vi "Main.vi"(11 "Module Admin":refnum<class "Delacor_lib_QMH_Module Admin.lvclass">) -> ()   [LabVIEW 2021, in "SCOPE.lvlib"]
doc: "This template is based off of the Queued Message Handler design pattern and the Queued Message Handler project template that ships with LabVIEW.\n\nThe main difference is that the queue is private to this module and communication between modules is performed via Broadcast and Request events.\n\nRequest events are wrapped in public API methods and are handled in the Event Handling Loop (EHL) of this VI. Any module can register for Broadcast events sent by this module. The EHL generates messages based on user interface actions.\n\nThe Message Handling Loop (MHL) processes messages generated by the EHL, or by other messages. The messages are string values, so new messages can be added easily to the Message Cases case structure in the MHL. Each message cluster can also provide an optional value for Message Data, which is a variant that can be converted to whatever message-specific data is required.\n_____\nBased on Delacor QMH Project Template 5.0.0.82.\n\n<b>Note:</b> This VI was modified by the <b>Validate DQMH Module</b> tool to add a 'Panel Hidden' status updated broadcast to the Panel Close? event when External Launch = TRUE.\n\n<b>Note:</b> This VI was modified by the <b>Validate DQMH Module</b> tool to add a call to the Error Reported VI at the end of the 'Exit' MHL frame.\n\n<b>Note:</b> This VI was modified by the <b>Validate DQMH Module</b> tool to wrap the FP.Open method in the module close code with a Conditional Disable Structure so it does not execute when the Main VI is running as a built EXE."
uses:
  SCOPE.lvlib
  <vilib>/Delacor/Delacor QMH/Libraries/Module Admin_class/Delacor_lib_QMH_Module Admin.lvclass
  Module Data--cluster.ctl
  <vilib>/Delacor/Delacor QMH/Libraries/Message Queue_class/Delacor_lib_QMH_Message Queue.lvclass/Delacor_lib_QMH_Message Queue.ctl
  Stop Argument--cluster.ctl
  <vilib>/Delacor/Delacor QMH/Libraries/Module Admin_class/Delacor_lib_QMH_Module Admin.lvclass/Delacor_lib_QMH_Module Admin.ctl
  Simulation Argument--cluster.ctl
  Acquire Signal Argument--cluster.ctl
  Load in SubPane Argument--cluster.ctl
  UnLoad SubPane Argument--cluster.ctl
  <vilib>/Utility/miscctls.llb/LVPointTypeDef.ctl
  <vilib>/Delacor/Delacor QMH/Libraries/Message Queue_class/Delacor_lib_QMH_Enqueue Message (Single).vi
  <vilib>/Delacor/Delacor QMH/Libraries/Module Admin_class/Delacor_lib_QMH_Get External Launch.vi
  <vilib>/Utility/error.llb/Error Cluster From Error Code.vi
  <vilib>/ErrorRing/Error Ring.xnode
  <vilib>/Delacor/Delacor QMH/Libraries/Message Queue_class/Delacor_lib_QMH_Message Queue.lvclass
  Model/Model.lvlib
panel:
  in  "AcqTime":dbl=5.0
  out "ElapsedTime":dbl
  in  "Sim":bool
  out "WFM":dbl[](graph)
  in  "Acquire":bool
  out "Subpanel Ref":refnum<vi>
  out "ModuleName":string
  out "Sim?":bool
  in  "Simulate MHL Error":bool
  in  "Simulate EHL Error":bool
  out "error out":errorcluster
  out "Status":string
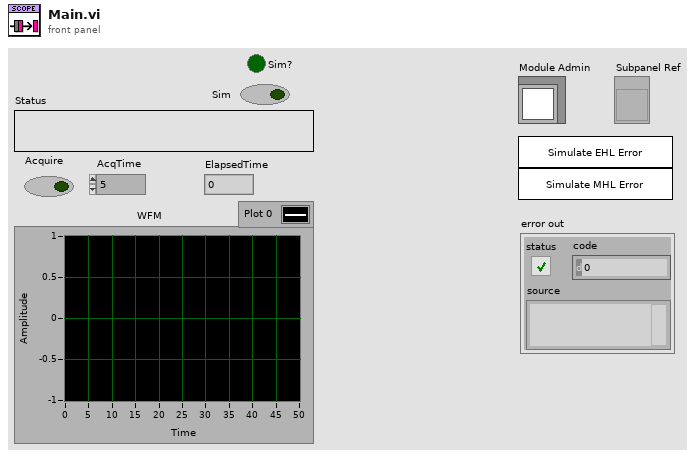
[diagram p1: front panel]
types:
  T1 = typedef "SCOPE.lvlib/Request Events--cluster.ctl" = cluster{"Stop Module":refnum<user-event>, "Show Panel":refnum<user-event>, "Hide Panel":refnum<user-event>, "Get Module Execution Status":refnum<user-event>, "Show Diagram":refnum<user-event>, "Simulation":refnum<user-event>, "Acquire Signal":refnum<user-event>, "Load in SubPane":refnum<user-event>, "UnLoad SubPane":refnum<user-event>}
  T2 = typedef "SCOPE.lvlib/Module Data--cluster.ctl" = cluster{"Status":string, "Sim":bool}
  T3 = enum32{"invalid lock state", "Not Locked", "Locked (No Password)", "Password-protected"}
  T4 = typedef "SCOPE.lvlib/Stop Argument--cluster.ctl" = cluster{"Origin":string, "Exit via Stop Module Req?":bool, "Wait for Module to stop?":bool}
  T5 = typedef "SCOPE.lvlib/Simulation Argument--cluster.ctl" = cluster{"Sim?":bool}
  T6 = typedef "SCOPE.lvlib/Acquire Signal Argument--cluster.ctl" = cluster{"Rate":i32, "AcqTime":dbl}
  T7 = typedef "SCOPE.lvlib/Load in SubPane Argument--cluster.ctl" = cluster{"Subpanel Ref":refnum<vi>}
  T8 = typedef "SCOPE.lvlib/UnLoad SubPane Argument--cluster.ctl" = cluster{"Subpanel Ref":refnum<vi>}
  T9 = typedef "LVPointTypeDef.ctl" = cluster{"Horizontal":i16, "Vertical":i16}
  T10 = enum32{"Invalid", "Standard", "Closed", "Hidden", "Minimized", "Maximized"}
  T11 = typedef "eventvkey.ctl" = enum16{"ASCII", "Enter", "Return", "Shift", "Ctrl", "Alt", "Cmd", "Opt", "Caps", "NumLock", "Clear", "Break", "Up", "Down", "Left", "Right", "Insert", "Delete", "Home", "End", "PageUp", "PageDown", "Escape", "Help", "Pause", "ScrollLock", "F1", "F2", "F3", "F4", "F5", "F6", "F7", "F8", "F9", "F10", "F11", "F12", "F13", "F14", "F15", "F16", "F17", "F18", "F19", "F20", "F21", "F22", "F23", "F24", "Play", "VolumeUp", "VolumeDown", "Mute", "Two Byte Char"}
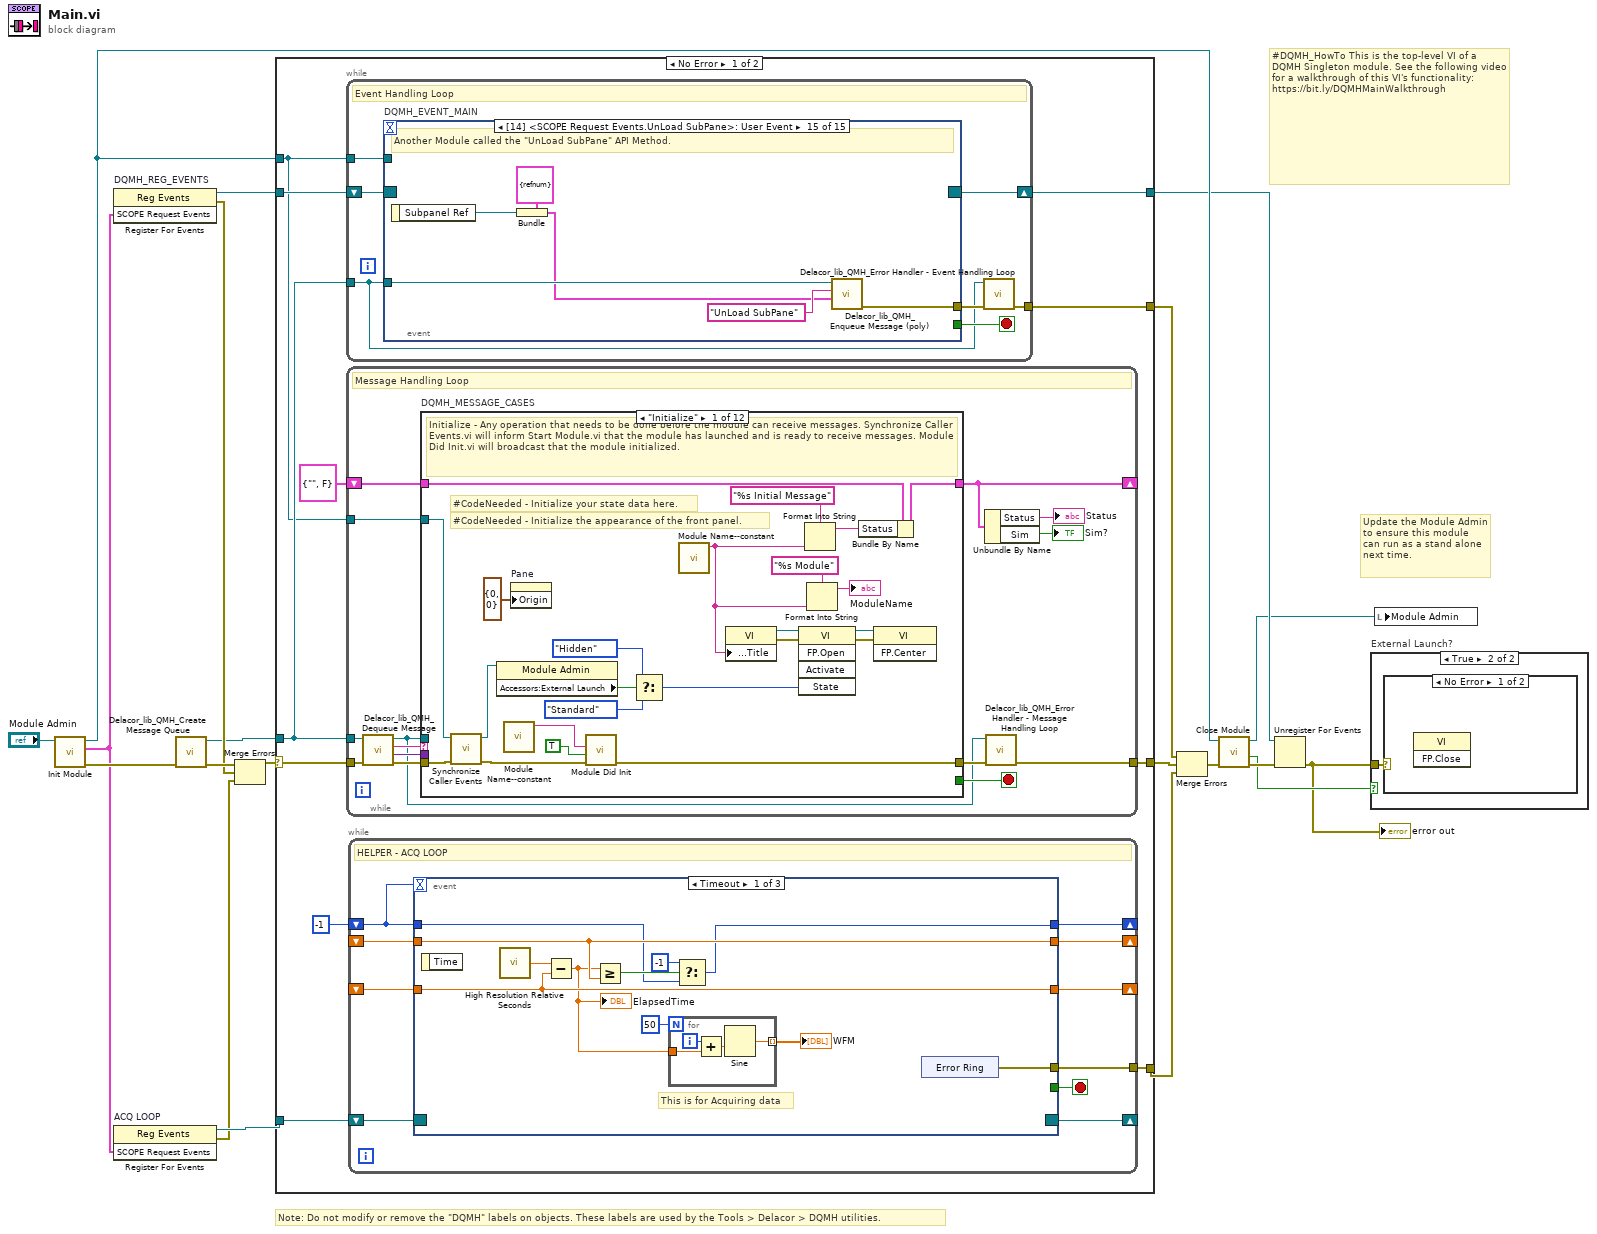
[diagram p0: block diagram]
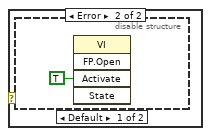
[diagram p3: hidden frame]
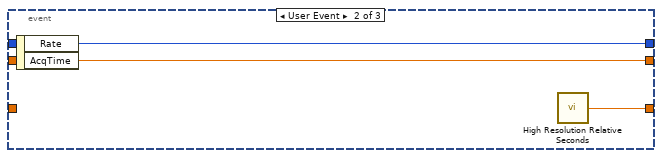
[diagram p5: hidden frame]
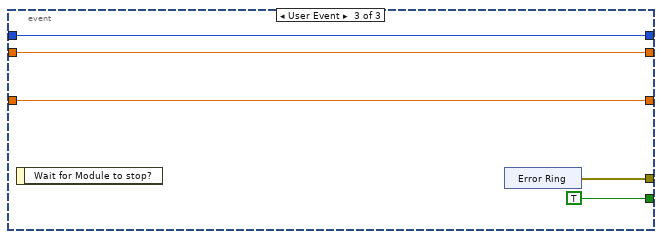
[diagram p6: hidden frame]
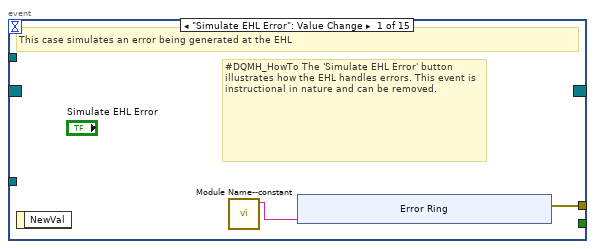
[diagram p7: hidden frame]
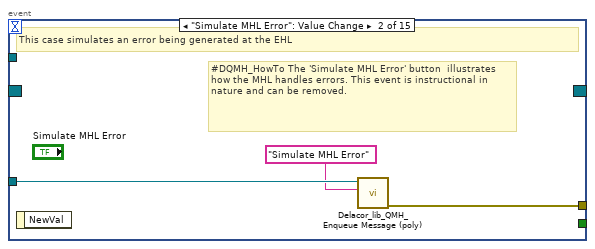
[diagram p8: hidden frame]
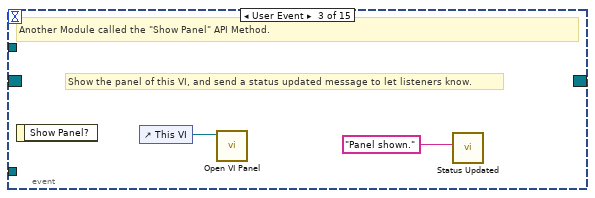
[diagram p9: hidden frame]
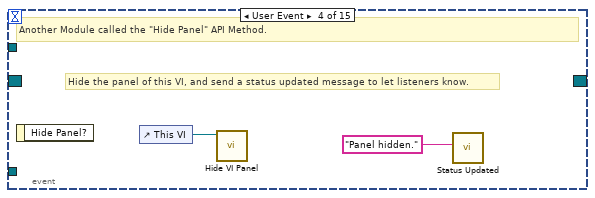
[diagram p10: hidden frame]
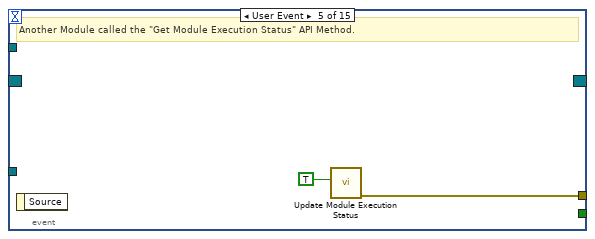
[diagram p11: hidden frame]
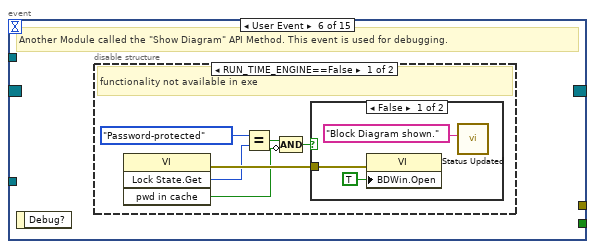
[diagram p12: hidden frame]
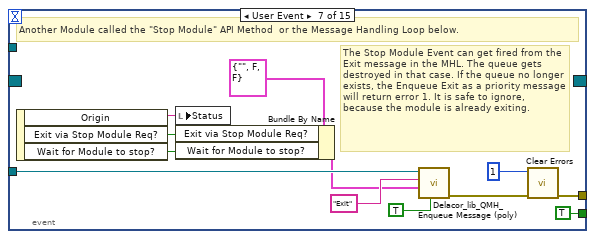
[diagram p15: hidden frame]
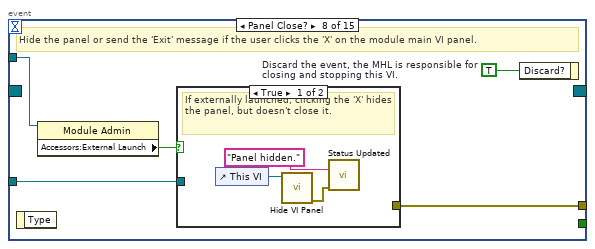
[diagram p16: hidden frame]
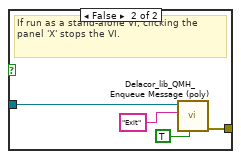
[diagram p17: hidden frame]
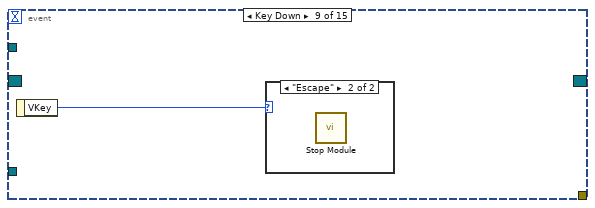
[diagram p18: hidden frame]
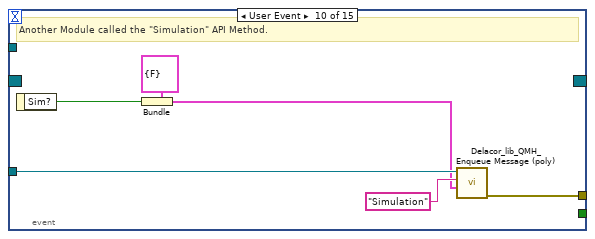
[diagram p20: hidden frame]
diagram:
  # "#DQMH_HowTo This is the top-level VI of a DQMH Singleton module. See the following video for a walkthrough of this VI's functionality: https://bit.ly/DQMHMainWalkthrough"
  # "Note: Do not modify or remove the \"DQMH\" labels on objects. These labels are used by the Tools > Delacor > DQMH utilities."
  # "Update the Module Admin to ensure this module can run as a stand alone next time."
  n1 = call "Init Module.vi"("Singleton Module Admin in"="Module Admin") -> ("error out"=w19:errorcluster, "SCOPE Request Events"=w5:T1, "Singleton Module Admin out"=w12:refnum<class "Delacor_lib_QMH_Module Admin.lvclass">)  [unwired: 8 in]
  n2 = register-events "DQMH_REG_EVENTS"(w5) -> (reference out=w10:refnum<event-registration>, error out=w13:errorcluster)  [unwired: 2 in]
  n3 = register-events "ACQ LOOP"(w5) -> (reference out=w4:refnum<event-registration>, error out=w2:errorcluster)  [unwired: 2 in]
  n4 = call <vilib>:"Delacor_lib_QMH_Create Message Queue.vi"("error in"=w19) -> ("error out"=w15:errorcluster, "Message Queue"=w9:refnum<class "Delacor_lib_QMH_Message Queue.lvclass">)  [unwired: 9 in]
  n5 = Merge Errors(w15, w13, w2) -> (w14:errorcluster)
  n6 = case shown="No Error" w14 {
    selector: w14 -> [w29 w298]
    tunnel: [w31 w296] -> w20
    tunnel: [w28 w303] -> w11
    tunnel: w10 -> [w26 w303]
    tunnel: w9 -> [w25 w297]
    tunnel: [w30 _] -> w17
    tunnel: w12 -> [w24 w299]
    tunnel: w4 -> [w23 _]
    tunnel: [w22 _] -> w3
    frame No Error {
      n7 = while {
        tunnel: w25 -> [w67]
        shift-right: [w70] -> w28
        shift-left: w26 -> [w71]
        tunnel: [w72] -> w30
        tunnel: w24 -> [w68]
        stop <- w69 stop-if-true
        # "Event Handling Loop"
        n8 = event "DQMH_EVENT_MAIN" shown="[14] <SCOPE Request Events.UnLoad SubPane>: User Event" {
          selector: w71 -> [_ _ _ _ _ _ _ _ _ _ _ _ _ _ _]
          dyn-events: [_ _ _ _ _ _ _ _ _ _ _ _ _ _ _] -> w70
          timeout: _ -> [_ _ _ _ _ _ _ _ _ _ _ _ _ _ _]
          tunnel: [_ _ _ _ _ _ TRUE ("Discard?") _ _ _ _ _ _ _ _] -> w69
          tunnel: w67 -> [_ w84 _ _ _ _ w108 w115 _ w131 w138 _ _ w152 w158]
          tunnel: [w75 w85 _ _ w91 _ w111 w117 _ w126 w133 w144 w146 w147 w153] -> w73
          tunnel: w68 -> [_ _ _ _ _ _ _ w114 _ _ _ _ _ _ _]
          event "Simulate EHL Error": Value Change {
            # "#DQMH_HowTo The 'Simulate EHL Error' button  illustrates how the EHL handles errors. This event is instructional in nature and can be removed."
            # "This case simulates an error being generated at the EHL"
            n9 = event-data() -> ()  [unwired: 1 in, 1 out]
            n10 = call "Module Name--constant.vi"() -> ("Module Name"=w74:string)  [unwired: 11 in]
            n11 = xnode ("Error Ring")("parameter 0"=w74) -> ("error out"=w75:errorcluster)
          }
          event "Simulate MHL Error": Value Change {
            # "#DQMH_HowTo The 'Simulate MHL Error' button  illustrates how the MHL handles errors. This event is instructional in nature and can be removed."
            # "This case simulates an error being generated at the EHL"
            n12 = event-data() -> ()  [unwired: 1 in, 1 out]
            n13 = call-poly <vilib>:"Delacor_lib_QMH_Enqueue Message (poly).vi"("Message"="Simulate MHL Error", "Message Queue in"=w84) -> ("error out"=w85:errorcluster)  [unwired: 8 in, 1 out]
          }
          event User Event {
            # "Show the panel of this VI, and send a status updated message to let listeners know."
            # "Another Module called the \"Show Panel\" API Method."
            n14 = event-data() -> ()  [unwired: 1 in, 1 out]
            n15 = control-ref of="This VI"() -> (w87:refnum<vi>)
            n16 = call "Open VI Panel.vi"("VI"=w87) -> ()  [unwired: 10 in, 1 out]
            n17 = call "Status Updated.vi"("Status"="Panel shown." ("format string")) -> ()  [unwired: 10 in, 1 out]
          }
          event User Event {
            # "Hide the panel of this VI, and send a status updated message to let listeners know."
            # "Another Module called the \"Hide Panel\" API Method."
            n18 = event-data() -> ()  [unwired: 1 in, 1 out]
            n19 = control-ref of="This VI"() -> (w89:refnum<vi>)
            n20 = call "Hide VI Panel.vi"("VI"=w89) -> ()  [unwired: 10 in, 1 out]
            n21 = call "Status Updated.vi"("Status"="Panel hidden." ("format string")) -> ()  [unwired: 10 in, 1 out]
          }
          event User Event {
            # "Another Module called the \"Get Module Execution Status\" API Method."
            n22 = event-data() -> ()  [unwired: 1 in, 1 out]
            n23 = call "Update Module Execution Status.vi"("Running?"=TRUE) -> ("error out"=w91:errorcluster)  [unwired: 10 in]
          }
          event User Event {
            # "Another Module called the \"Show Diagram\" API Method. This event is used for debugging."
            n24 = event-data() -> ()  [unwired: 1 in, 1 out]
            n25 = disable-structure "Conditional Disable Structure" shown="RUN_TIME_ENGINE==False" {
              frame condition #0 (active) {
                # "functionality not available in exe"
                n26 = invoke on="Invoke Node" class="VI" method="Lock State.Get"() -> (error out=w97:errorcluster, "Get Lock State"=w96:T3, "pwd in cache"=w93:bool)  [unwired: 4 in, 1 out]
                n27 = Equal?(x=T3."Password-protected", y=w96) -> (x = y?=w94:bool)
                n28 = Compound Arithmetic op=AND(w94, invert w93) -> (w92:bool)
                n29 = case shown="False" w92 {
                  tunnel: w97 -> [w100 _]
                  frame False {
                    n30 = property on="Property Node" class="VI"(error in=w100, "BDWin.Open"=TRUE ("Block Diagram Window:Open")) -> ()  [unwired: 1 in, 2 out]
                    n31 = call "Status Updated.vi"("Status"="Block Diagram shown." ("format string")) -> ()  [unwired: 10 in, 1 out]
                  }
                  frame True {
                    # "Password-protected VI, and the password is not in the cache. Do not show the diagram."
                  }
                }
              }
              frame condition #1 {
              }
            }
          }
          event User Event {
            # "The Stop Module Event can get fired from the Exit message in the MHL. The queue gets destroyed in that case. If the queue no longer exists, the Enqueue Exit as a priority message will return error 1. It is safe to ignore, because the module is already exiting."
            # "Another Module called the \"Stop Module\" API Method  or the Message Handling Loop below."
            n32 = event-data() -> ("Origin"=w107:string, "Exit via Stop Module Req?"=w103:bool, "Wait for Module to stop?"=w102:bool)  [unwired: 1 in]
            n33 = local write "Status"(w107) -> ()
            n34 = Bundle By Name(cluster=T4 {"Origin"="", "Exit via Stop Module Req?"=FALSE, "Wait for Module to stop?"=FALSE} ("Stop Argument"), "Exit via Stop Module Req?"=w103, "Wait for Module to stop?"=w102) -> (w101:T4)
            n35 = call-poly <vilib>:"Delacor_lib_QMH_Enqueue Message (poly).vi"("Priority Message? (F)"=TRUE, "Message Data"=w101, "Message"="Exit", "Message Queue in"=w108) -> ("error out"=w112:errorcluster)  [unwired: 6 in, 1 out]
            n36 = call <vilib>:"Clear Errors.vi"("error in (no error)"=w112, "specific error code to clear (0: all)"=1) -> ("error out"=w111:errorcluster)  [unwired: 4 in, 1 out]
          }
          event Panel Close? {
            w116 = TRUE  # Discard the event, the MHL is responsible for closing and stopping this VI.
            # "Hide the panel or send the 'Exit' message if the user clicks the 'X' on the module main VI panel."
            n37 = event-data() -> ()  [unwired: 1 in, 1 out]
            n38 = property on="Property Node" class="Module Admin"(reference=w114) -> ("Accessors:External Launch"=w113:bool)  [unwired: 1 in, 2 out]
            n39 = case shown="True" w113 {
              tunnel: w115 -> [_ w123]
              tunnel: [_ w124] -> w117
              frame True {
                # "If externally launched, clicking the 'X' hides the panel, but doesn't close it."
                n40 = control-ref of="This VI"() -> (w120:refnum<vi>)
                n41 = call "Hide VI Panel.vi"("VI"=w120) -> ("error out"=w118:errorcluster)  [unwired: 10 in]
                n42 = call "Status Updated.vi"("error in (no error)"=w118, "Status"="Panel hidden.") -> ()  [unwired: 9 in, 1 out]
              }
              frame False {
                # "If run as a stand-alone VI, clicking the panel 'X' stops the VI."
                n43 = call-poly <vilib>:"Delacor_lib_QMH_Enqueue Message (poly).vi"("Priority Message? (F)"=TRUE, "Message"="Exit", "Message Queue in"=w123) -> ("error out"=w124:errorcluster)  [unwired: 7 in, 1 out]
              }
            }
            n44 = event-data ("Event Filter Node")("Discard?"=w116) -> ()  [unwired: 1 in, 1 out]
          }
          event Key Down {
            n45 = event-data() -> ("VKey"=w125:T11)  [unwired: 1 in]
            n46 = case shown="\"Escape\"" w125 {
              frame Default {
              }
              frame "Escape" {
                n47 = call "Stop Module.vi"() -> ()  [unwired: 11 in, 1 out]
              }
            }
          }
          event User Event {
            # "Another Module called the \"Simulation\" API Method."
            n48 = event-data() -> ("Sim?"=w127:bool)  [unwired: 1 in]
            n49 = Bundle(cluster=T5 {"Sim?"=FALSE} ("Simulation Argument"), "Sim?"=w127) -> (w128:T5)
            n50 = call-poly <vilib>:"Delacor_lib_QMH_Enqueue Message (poly).vi"("Message Data"=w128, "Message"="Simulation", "Message Queue in"=w131) -> ("error out"=w126:errorcluster)  [unwired: 7 in, 1 out]
          }
          event User Event {
            # "Another Module called the \"Acquire Signal\" API Method."
            n51 = event-data() -> ("Rate"=w134:i32, "AcqTime"=w132:dbl)  [unwired: 1 in]
            n52 = Bundle(cluster=T6 {"Rate"=0, "AcqTime"=20.0} ("Acquire Signal Argument"), "Rate"=w134, "AcqTime"=w132) -> (w135:T6)
            n53 = call-poly <vilib>:"Delacor_lib_QMH_Enqueue Message (poly).vi"("Message Data"=w135, "Message"="Acquire Signal", "Message Queue in"=w138) -> ("error out"=w133:errorcluster)  [unwired: 7 in, 1 out]
          }
          event "Acquire": Value Change {
            n54 = event-data() -> ()  [unwired: 1 in, 1 out]
            n55 = Select(t=10, s="Acquire", f=-1) -> (s? t:f=w139:i32)
            n56 = call "Acquire Signal.vi"("AcqTime"="AcqTime", "Rate"=w139) -> ("error out"=w144:errorcluster)  [unwired: 9 in]
          }
          event "Sim": Value Change {
            n57 = event-data() -> ()  [unwired: 1 in, 1 out]
            n58 = call "Simulation.vi"("Sim?"="Sim") -> ("error out"=w146:errorcluster)  [unwired: 10 in]
          }
          event User Event {
            # "Another Module called the \"Load in SubPane\" API Method."
            n59 = event-data() -> ("Subpanel Ref"=w148:refnum<vi>)  [unwired: 1 in]
            n60 = Bundle(cluster=T7 {"Subpanel Ref"=refnum} ("Load in SubPane Argument"), "Subpanel Ref"=w148) -> (w149:T7)
            n61 = call-poly <vilib>:"Delacor_lib_QMH_Enqueue Message (poly).vi"("Message Data"=w149, "Message"="Load in SubPane", "Message Queue in"=w152) -> ("error out"=w147:errorcluster)  [unwired: 7 in, 1 out]
          }
          event User Event {
            # "Another Module called the \"UnLoad SubPane\" API Method."
            n62 = event-data() -> ("Subpanel Ref"=w154:refnum<vi>)  [unwired: 1 in]
            n63 = Bundle(cluster=T8 {"Subpanel Ref"=refnum} ("UnLoad SubPane Argument"), "Subpanel Ref"=w154) -> (w155:T8)
            n64 = call-poly <vilib>:"Delacor_lib_QMH_Enqueue Message (poly).vi"("Message Data"=w155, "Message"="UnLoad SubPane", "Message Queue in"=w158) -> ("error out"=w153:errorcluster)  [unwired: 7 in, 1 out]
          }
        }
        n65 = call-dynamic "Delacor_lib_QMH_Error Handler - Event Handling Loop.vi"("error in"=w73, "Message Queue in"=w67) -> ("dup error in"=w72:errorcluster)  [unwired: 8 in, 1 out]
      }
      n66 = while {
        tunnel: w25 -> [w164]
        shift-right: [w161] -> _
        shift-left: T2 {"Status"="", "Sim"=FALSE} ("Data Cluster") -> [w168]
        tunnel: w29 -> [w171]
        tunnel: [w169] -> w31
        tunnel: w24 -> [w162]
        stop <- w167 stop-if-true
        # "Message Handling Loop"
        n67 = call-dynamic "Delacor_lib_QMH_Dequeue Message.vi"("error in"=w171, "Message Queue in"=w164) -> ("error out"=w170:errorcluster, "Message Data"=w165:variant, "Message"=w166:string, "Message Queue out"=w163:refnum<class "Delacor_lib_QMH_Message Queue.lvclass">)  [unwired: 6 in]
        n68 = case "DQMH_MESSAGE_CASES" shown="\"Initialize\"" w166 {
          selector: w166 -> [_ _ w204 _ _ _ _ _ _ _ _ w283]
          tunnel: w163 -> [_ _ _ _ _ _ _ _ _ w251 w275 _]
          tunnel: w170 -> [w193 w197 w211 w216 w224 w231 w234 w236 w241 w258 w281 w285]
          tunnel: [w191 w197 w209 w212 w222 w229 w233 w236 w240 w254 w278 w286] -> w172
          tunnel: w168 -> [w184 w196 w210 w215 w223 w230 w232 w235 w238 w253 w274 w284]
          tunnel: [w183 w196 w205 w215 w223 w230 w232 w235 w238 w253 w274 w284] -> w161
          tunnel: [_ _ _ _ _ _ _ _ _ _ w273 _] -> w167
          tunnel: w165 -> [_ _ w208 w214 w221 w228 _ _ _ w252 w272 _]
          tunnel: w162 -> [w185 _ _ _ _ _ _ _ _ w250 w267 _]
          frame "Initialize" {
            # "#CodeNeeded - Initialize the appearance of the front panel."
            # "#CodeNeeded - Initialize your state data here."
            # "Initialize - Any operation that needs to be done before the module can receive messages. Synchronize Caller Events.vi will inform Start Module.vi that the module has launched and is ready to receive messages. Module Did Init.vi will broadcast that the module initialized."
            n69 = call "Synchronize Caller Events.vi"("error in (no error)"=w193, "Singleton Module Admin in"=w185) -> ("error out"=w192:errorcluster, "Singleton Module Admin out"=w180:refnum<class "Delacor_lib_QMH_Module Admin.lvclass">)  [unwired: 8 in]
            n70 = property on="Property Node" class="Module Admin"(reference=w180) -> ("Accessors:External Launch"=w189:bool)  [unwired: 1 in, 2 out]
            n71 = call "Module Name--constant.vi"() -> ("Module Name"=w181:string)  [unwired: 11 in]
            n72 = property on="Pane" class="Pane"("Origin"=T9 {"Horizontal"=0, "Vertical"=0}) -> ()  [unwired: 2 in, 2 out]
            n73 = call "Module Did Init.vi"("error in (no error)"=w192, "Initialized?"=TRUE, "Origin"=w181) -> ("error out"=w191:errorcluster)  [unwired: 8 in]
            n74 = Select(t=T10."Hidden" ("State"), s=w189, f=T10."Standard" ("State")) -> (s? t:f=w186:T10)
            n75 = call "Module Name--constant.vi"() -> ("Module Name"=w176:string)  [unwired: 11 in]
            n76 = property on="Property Node" class="VI"("Front Panel.Title"=w176) -> (reference out=w190:refnum<vi>, error out=w195:errorcluster)  [unwired: 2 in]
            n77 = invoke on="Invoke Node" class="VI" method="FP.Open"(reference=w190, error in=w195, "State"=w186) -> (reference out=w173:refnum<vi>, error out=w194:errorcluster)  [unwired: 2 in, 3 out]
            n78 = Format Into String(format string="%s Initial Message" ("Initial Message"), w176) -> (resulting string=w178:string)  [unwired: 2 in, 1 out]
            n79 = Format Into String(format string="%s Module", w176) -> (resulting string=→"ModuleName":string)  [unwired: 2 in, 1 out]
            n80 = Bundle By Name(cluster=w184, "Status"=w178) -> (w183:T2)
            n81 = invoke on="Invoke Node" class="VI" method="FP.Center"(reference=w173, error in=w194) -> ()  [unwired: 1 in, 3 out]
          }
          frame "--- Module Specific ---" {
            # "Separator -- The following cases handle messages specific to this Module."
          }
          frame "Simulation" {
            # "This will change Module into Simulation Mode"
            n82 = Variant To Data(error in=w211, type=T5 {"Sim?"=FALSE} ("Simulation Argument"), Variant=w208) -> (data=w206:T5, error out=w209:errorcluster)
            n83 = Unbundle By Name(w206) -> ("Sim?"=w203:bool)
            n84 = Select(t="True", s=w203, f="False") -> (s? t:f=w199:string)
            n85 = Format Into String(format string="%s: %s", w204, w199) -> (resulting string=w198:string)  [unwired: 2 in, 1 out]
            n86 = Bundle By Name(cluster=w210, "Status"=w198, "Sim"=w203) -> (w205:T2)
          }
          frame "Acquire Signal" {
            # "This event is for Helper Loop"
            # "This will acquires signal at CH0"
            n87 = Variant To Data(error in=w216, type=T6 {"Rate"=0, "AcqTime"=20.0} ("Acquire Signal Argument"), Variant=w214) -> (error out=w212:errorcluster)  [unwired: 1 out]
          }
          frame "Load in SubPane" {
            n88 = Variant To Data(error in=w224, type=T7 {"Subpanel Ref"=refnum} ("Load in SubPane Argument"), Variant=w221) -> (data=w219:T7, error out=w222:errorcluster)
            n89 = Unbundle By Name(w219) -> ("Subpanel Ref"=w217:refnum<vi>)
            "Subpanel Ref" <- w217
            n90 = control-ref of="This VI"() -> (w218:refnum<vi>)
            n91 = call "Insert SubPanl.vi"("VI Ref"=w218, "Subpanel Ref"=w217) -> ()  [unwired: 9 in, 1 out]
          }
          frame "UnLoad SubPane" {
            n92 = Variant To Data(error in=w231, type=T8 {"Subpanel Ref"=refnum} ("UnLoad SubPane Argument"), Variant=w228) -> (data=w226:T8, error out=w229:errorcluster)
            n93 = Unbundle By Name(w226) -> ("Subpanel Ref"=w225:refnum<vi>)
            n94 = call "Remove SubPanel.vi"("Subpanel Ref"=w225) -> ()  [unwired: 10 in, 1 out]
          }
          frame "---Copy This Frame---" {
            # "Duplicate this frame when creating new messages.  Change this comment in the duplicated frame to describe this message."
            n95 = Merge Errors(w234) -> (w233:errorcluster)
          }
          frame "--- Exit and Error Handling---" {
            # "Separator - The following cases handle errors and exit messages."
          }
          frame "Simulate MHL Error" {
            # "#DQMH_HowTo The 'Simulate MHL Error' button  illustrates how the MHL handles errors. This event is instructional in nature and can be removed."
            # "Simulate an error occurring at the MHL"
            n96 = call "Module Name--constant.vi"() -> ("Module Name"=w237:string)  [unwired: 11 in]
            n97 = xnode ("Error Ring")("parameter 0"=w237) -> ("error out"=w239:errorcluster)
            n98 = Merge Errors(w241, w239) -> (w240:errorcluster)
          }
          frame "Error" {
            # "#CodeRecommended - If you ever change the name of this \"Error\" message, you'll need to update the name in the Check Loop Error.vi as well."
            # "#CodeRecommended - If the module is running in standalone mode (External Launch = FALSE), this code will pop up an error dialog and call the 'Exit' message if an error occurs. Add more fine-grained error handling here."
            # "Error - Check the error message data and respond accordingly. This message is sent by the \"Error Handler\" VIs at the end of each loop in this application."
            n99 = property on="Property Node" class="Module Admin"(reference=w250) -> ("Accessors:External Launch"=w249:bool)  [unwired: 1 in, 2 out]
            n100 = Variant To Data(error in=w258, type=errorcluster {"status"=FALSE, "code"=0, "source"=""} ("error constant"), Variant=w252) -> (data=w259:errorcluster, error out=w256:errorcluster)
            n101 = call "Error Reported.vi"("Error"=w259) -> ()  [unwired: 10 in, 1 out]
            n102 = case shown="False" w249 {
              tunnel: [w264 _] -> w255
              tunnel: w251 -> [w262 _]
              tunnel: w259 -> [w263 _]
              frame False {
                # "If the module is running standalone, then pop up an error dialog and call the \"Exit\" message."
                n103 = call <vilib>:"Simple Error Handler.vi"("error in (no error)"=w263) -> ()  [unwired: 4 in, 5 out]
                n104 = call-poly <vilib>:"Delacor_lib_QMH_Enqueue Message (poly).vi"("Priority Message? (F)"=TRUE, "Message"="Exit", "Message Queue in"=w262) -> ("error out"=w264:errorcluster)  [unwired: 7 in, 1 out]
              }
              frame True {
                # "If the module was launched externally, calling the Error Reported broadcast VI is the only action performed by the \"Error\" message. The module's caller can then process the error appropriately."
              }
            }
            n105 = Merge Errors(w256, w255) -> (w254:errorcluster)
            n106 = local write "error out"(w254) -> ()
          }
          frame "Exit" {
            w271 = 91  # 91: not all Exit messages will have an argument
            w273 = TRUE  # Stop the VI
            # "Release the message queue reference"
            # "Exit - Exit the application."
            n107 = Variant To Data(error in=w281, type=T4 {"Origin"="", "Exit via Stop Module Req?"=FALSE, "Wait for Module to stop?"=FALSE} ("Stop Argument"), Variant=w272) -> (data=w269:T4, error out=w277:errorcluster)
            n108 = call <vilib>:"Clear Errors.vi"("error in (no error)"=w277, "specific error code to clear (0: all)"=w271) -> ("error out"=w280:errorcluster)  [unwired: 4 in, 1 out]
            n109 = local read "Subpanel Ref"() -> (w265:refnum<vi>)
            n110 = control-ref of="This VI"() -> (w268:refnum<vi>)
            n111 = call "Remove SubPanel.vi"("Subpanel Ref"=w265) -> ("error out"=w266:errorcluster)  [unwired: 10 in]
            n112 = call-dynamic "Delacor_lib_QMH_Release Message Queue.vi"("error in"=w280, "Message Queue"=w275) -> ("error out"=w279:errorcluster)  [unwired: 9 in]
            n113 = call "Handle Exit.vi"("error in (no error)"=w266, "Stop Argument"=w269, "Admin in"=w267, "VI reference"=w268) -> ("error out"=w276:errorcluster)  [unwired: 6 in, 1 out]
            n114 = Merge Errors(w279, w276) -> (w278:errorcluster)
            n115 = call "Error Reported.vi"("Error"=w278) -> ()  [unwired: 10 in, 1 out]
          }
          frame Default {
            # "'Default' case only runs if there is a message that isn't defined in any of the other cases.  Output a programming error."
            n116 = call "Module Name--constant.vi"() -> ("Module Name"=w282:string)  [unwired: 11 in]
            n117 = xnode ("Error Ring")("parameter 0"=w283, "parameter 1"=w282) -> ("error out"=w287:errorcluster)
            n118 = Merge Errors(w285, w287) -> (w286:errorcluster)
          }
        }
        n119 = Unbundle By Name(w161) -> ("Status"=→"Status":string, "Sim"=→"Sim?":bool)
        n120 = call-dynamic "Delacor_lib_QMH_Error Handler - Message Handling Loop.vi"("error in"=w172, "Message Queue in"=w163) -> ("dup error in"=w169:errorcluster)  [unwired: 8 in, 1 out]
      }
      n121 = while {
        shift-right: [w39] -> _
        shift-left: w23 -> [w41]
        tunnel: [w38] -> w22
        shift-right: [w36] -> _
        shift-left: -1 -> [w37]
        shift-right: [w35] -> _
        shift-left: _ -> [w34]
        shift-right: [w33] -> _
        shift-left: _ -> [w32]
        stop <- w40 stop-if-true
        # "HELPER - ACQ LOOP"
        n122 = event shown="[0] Timeout" {
          selector: w41 -> [_ _ _]
          dyn-events: [_ _ _] -> w39
          timeout: w37 -> [_ _ _]
          tunnel: [_ _ TRUE] -> w40
          tunnel: [w52 _ w64] -> w38
          tunnel: w37 -> [w44 _ w63]
          tunnel: [w43 w58 w63] -> w36
          tunnel: [w47 w60 w62] -> w35
          tunnel: w34 -> [w47 _ w62]
          tunnel: [w48 w59 w61] -> w33
          tunnel: w32 -> [w48 _ w61]
          event Timeout {
            # "This is for Acquiring data"
            n123 = event-data() -> ()  [unwired: 1 in, 1 out]
            n124 = call <vilib>:"High Resolution Relative Seconds.vi"() -> ("relative seconds"=w49:dbl)
            n125 = Subtract(x=w49, y=w47) -> (x-y=w42:dbl)
            "ElapsedTime" <- w42
            n126 = Greater Or Equal?(x=w42, y=w48) -> (x >= y?=w46:bool)
            n127 = for {
              N: 50 -> [_]
              tunnel: [w56] -> w51 mode=indexing
              tunnel: w42 -> [w53]
              i -> [w55]
              n128 = Add(x=w55, y=w53) -> (x+y=w54:dbl)
              n129 = Sine(x=w54) -> (sin(x)=w56:dbl)
            }
            "WFM" <- w51
            n130 = Select(t=-1, s=w46, f=w44) -> (s? t:f=w43:i32)
            n131 = xnode ("Error Ring")() -> ("error out"=w52:errorcluster)
          }
          event User Event {
            n132 = event-data() -> ("Rate"=w58:i32, "AcqTime"=w59:dbl)  [unwired: 1 in]
            n133 = call <vilib>:"High Resolution Relative Seconds.vi"() -> ("relative seconds"=w60:dbl)
          }
          event User Event {
            n134 = event-data() -> ()  [unwired: 1 in, 1 out]
            n135 = xnode ("Error Ring")() -> ("error out"=w64:errorcluster)
          }
        }
      }
    }
    frame Error {
      # "Synchronize Caller Events.vi will inform Start Module.vi that the module has launched and will let the code calling Start Module.vi register for broadcasts and would permit the caller receive the broadcast that an error occurred at launch time."
      n136 = call-dynamic "Delacor_lib_QMH_Release Message Queue.vi"("error in"=w298, "Message Queue"=w297) -> ("error out"=w296:errorcluster)  [unwired: 9 in]
      n137 = call "Synchronize Caller Events.vi"("Singleton Module Admin in"=w299) -> ("error out"=w304:errorcluster)  [unwired: 9 in, 1 out]
      n138 = call "Module Name--constant.vi"() -> ("Module Name"=w302:string)  [unwired: 11 in]
      n139 = Format Into String(format string="An error occurred during initialization. %s is no longer running.", w302) -> (resulting string=w300:string)  [unwired: 2 in, 1 out]
      n140 = Merge Errors(w296, w304) -> (w305:errorcluster)
      n141 = call "Error Reported.vi"("Additional Information"=w300, "Error"=w305) -> ()  [unwired: 9 in, 1 out]
    }
  }
  n142 = Merge Errors(w17, w20, w3) -> (w16:errorcluster)
  n143 = call "Close Module.vi"("error in (no error)"=w16, "Module Admin in"=w12) -> ("error out"=w18:errorcluster, "External Launch"=w6:bool, "Module Admin out"=w7:refnum<class "Delacor_lib_QMH_Module Admin.lvclass">)  [unwired: 7 in]
  n144 = Unregister For Events(event registration refnum=w11, error in=w18) -> (error out=w1:errorcluster)
  "error out" <- w1
  n145 = case "External Launch?" shown="True" w6 {
    tunnel: w1 -> [_ w306]
    frame False {
    }
    frame True {
      n146 = case shown="No Error" w306 {
        frame No Error {
          n147 = invoke on="Invoke Node" class="VI" method="FP.Close"() -> ()  [unwired: 3 in, 3 out]
        }
        frame Error {
          n148 = disable-structure shown="Default" {
            frame condition #0 (active) {
              n149 = invoke class="VI" method="FP.Open"("Activate"=TRUE ("Activate?")) -> ()  [unwired: 4 in, 5 out]
            }
            frame condition #1 {
              # "Don't show panel on error if running inside a built EXE."
            }
          }
        }
      }
    }
  }
  n150 = local write "Module Admin"(w7) -> ()
